vi "Get Project Info.vi"(8 "error in (no error)":errorcluster, 11 "Project Inspector Base in":refnum<class "Project Inspector Base.lvclass">) -> (0 "error out":errorcluster, 1 "Path":path, 2 "Name":string, 3 "Project Inspector Base out":refnum<class "Project Inspector Base.lvclass">, 4 "Item Paths":path[](array[path]))   [LabVIEW 2017, in "Cobertura.lvlib" / "Project Inspector Base.lvclass"]
uses:
  Project Inspector Base.lvclass
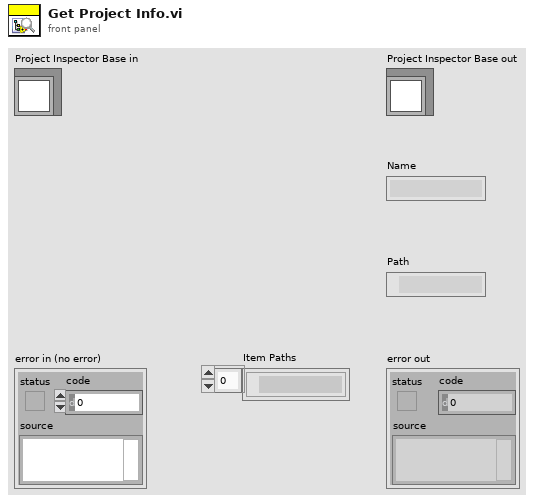
[diagram p1: front panel]
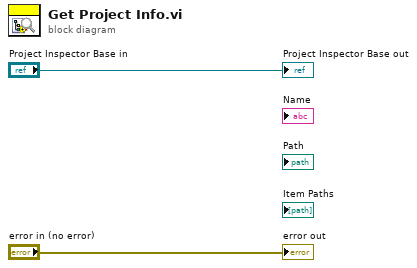
[diagram p0: block diagram]
diagram:
  "error out" <- "error in (no error)"
  "Project Inspector Base out" <- "Project Inspector Base in"
